vi "计算影像上的理论坐标.vi"(6 "Color":u32(colorbox)=16860, 8 "Y方向间隔":dbl=1.85 format="%#_13g", 9 "第一个坐标点":cluster{"X":dbl, "Y":dbl}, 10 "理论坐标位置输入":dbl[](array[numeric]), 11 "引用句柄输入":T1) -> (3 "理论影像坐标":cluster{dbl, "Numeric":dbl}[](array[cluster]))   [LabVIEW 2014]
uses:
  <vilib>/vision/Image Controls.llb/IMAQ Image.ctl
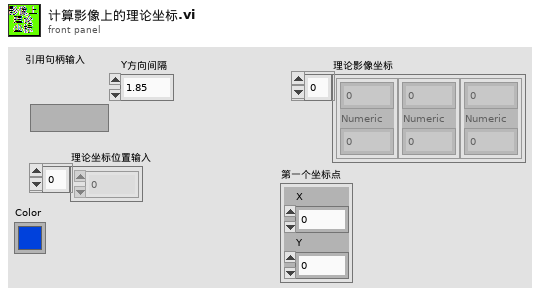
[diagram p1: front panel]
types:
  T1 = typedef "IMAQ Image.ctl" = refnum<image>
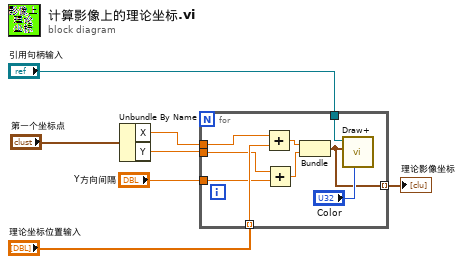
[diagram p0: block diagram]
diagram:
  n1 = Unbundle By Name("第一个坐标点") -> ("X"=w2:dbl, "Y"=w1:dbl)
  n2 = for {
    tunnel: "引用句柄输入" -> [w16]
    tunnel: w1 -> [w9]
    tunnel: "理论坐标位置输入" -> [w13] mode=indexing
    tunnel: w2 -> [w15]
    tunnel: [w11] -> w5 mode=indexing
    tunnel: "Y方向间隔" -> [w8]
    n3 = Add(x=w15, y=w13) -> (x+y=w14:dbl)
    n4 = Add(x=w9, y=w8) -> (x+y=w10:dbl)
    n5 = Bundle(w14, w10) -> (w11:cluster{dbl, dbl})  [unwired: 1 in]
    n6 = call "Draw+.vi"("Color"="Color", "input cluster"=w11, "Image In"=w16) -> ()  [unwired: 3 in, 1 out]
  }
  "理论影像坐标" <- w5
